vi "测试-读取txt文本.vi"() -> ()   [LabVIEW 2021]
panel:
  out "selected path":path caption="所选路径"
  out "显示":string
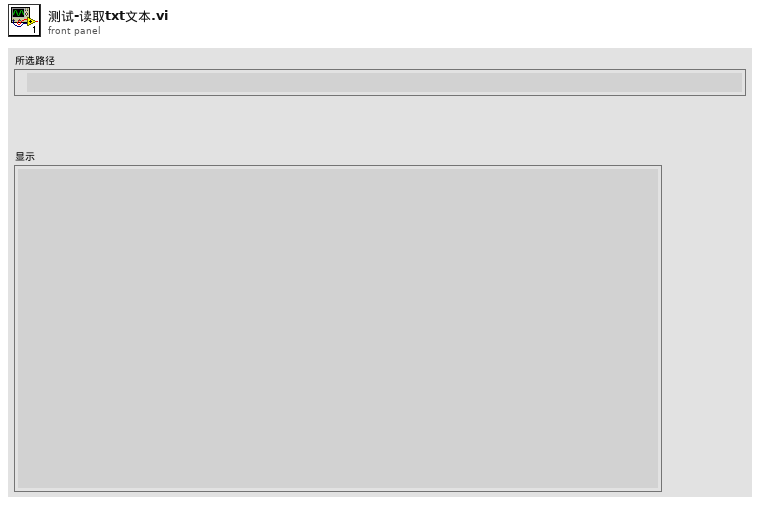
[diagram p1: front panel]
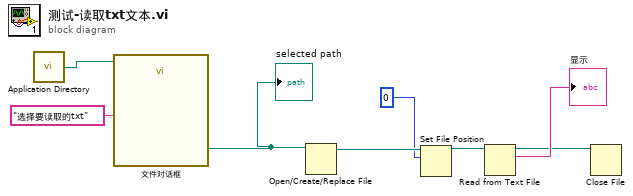
[diagram p0: block diagram]
diagram:
  n1 = call <vilib>:"Application Directory.vi"() -> ("Application Directory"=w6:path)
  n2 = call "文件对话框"("start path"=w6, "prompt"="选择要读取的txt") -> ("selected path"=w8:path)  [unwired: 10 in, 3 out]
  "selected path" <- w8
  n3 = Open/Create/Replace File(file path (use dialog)=w8) -> (refnum out=w5:refnum<file>)  [unwired: 5 in, 2 out]
  n4 = Set File Position(offset (in bytes) (0)=i64 0 ("偏移量（字节）（0）"), refnum=w5) -> (refnum out=w3:refnum<file>)  [unwired: 2 in, 1 out]
  n5 = Read from Text File(file (use dialog)=w3) -> (refnum out=w1:refnum<file>, text=→"显示":string)  [unwired: 3 in, 2 out]
  n6 = Close File(refnum=w1) -> ()  [unwired: 1 in, 2 out]
